vi "Source Current.vi"(7 "Channel Lists":string[](array[string]), 8 "error in (no error)":errorcluster, 10 "current level":dbl format="%_6p", 11 "Instrument Sessions In":refnum<k15>[](array[refnum])) -> (0 "error out":errorcluster, 1 "current measurements":dbl[][](array[numeric]), 2 "voltage measurements":dbl[][](array[numeric]), 3 "Instrument Sessions Out":refnum<k15>[](array[refnum]))   [LabVIEW 2013]
uses:
  <instrlib>/niDCPower/nidcpower.llb/niDCPower Wait For Event - Event.ctl
panel:
  out "Compliance":bool[](array[boolean])
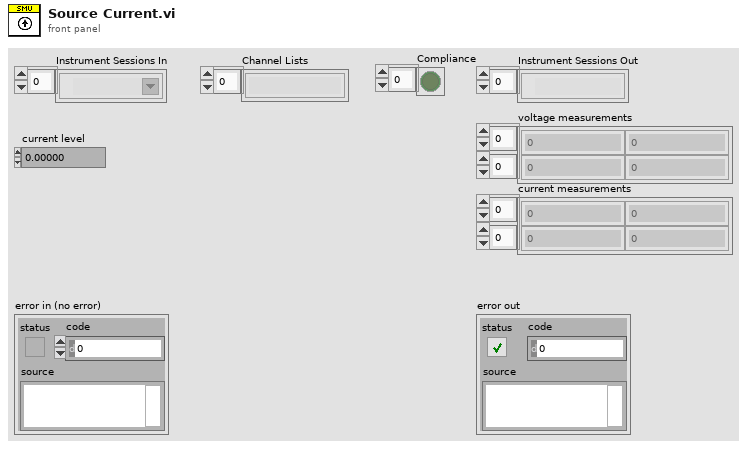
[diagram p1: front panel]
types:
  T1 = typedef "niDCPower Wait For Event - Event.ctl" = i32
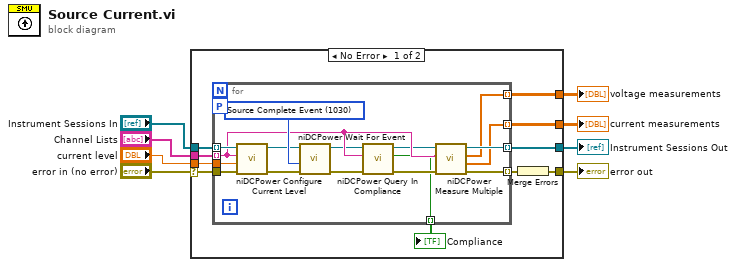
[diagram p0: block diagram]
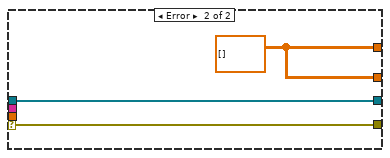
[diagram p2: hidden frame]
diagram:
  n1 = case shown="No Error" "error in (no error)" {
    selector: "error in (no error)" -> [w12 w36]
    tunnel: [w17 w36] -> w8
    tunnel: "Instrument Sessions In" -> [w16 w37]
    tunnel: "Channel Lists" -> [w15 _]
    tunnel: [w14 w37] -> w5
    tunnel: "current level" -> [w13 _]
    tunnel: [w11 w35] -> w2
    tunnel: [w10 w35] -> w1
    frame No Error {
      n2 = for {
        tunnel: w16 -> [w34] mode=indexing
        tunnel: w15 -> [w23] mode=indexing
        tunnel: [w28] -> w14 mode=indexing
        tunnel: [w27] -> w18 mode=indexing
        tunnel: w13 -> [w33]
        tunnel: w12 -> [w32]
        tunnel: [w25] -> w11 mode=indexing
        tunnel: [w26] -> w10 mode=indexing
        tunnel: [w19] -> w9 mode=indexing
        workers-P: _ -> [_]
        w30 = T1 1030 items=["Source Complete Event"=1030, "Measure Complete Event"=1031, "Sequence Iteration Complete Event"=1032, "Sequence Engine Done Event"=1033, "Pulse Complete Event"=1051, "Ready For Pulse Trigger Event"=1052] ("event")
        n3 = call <instrlib>:"niDCPower Configure Current Level.vi"("error in (no error)"=w32, "current level"=w33, "channel name"=w23, "instrument handle"=w34) -> ("error out"=w31:errorcluster, "instrument handle out"=w29:refnum<k15>)  [unwired: 6 in]
        n4 = call <instrlib>:"niDCPower Wait For Event.vi"("error in (no error)"=w31, "event"=w30, "instrument handle"=w29) -> ("error out"=w24:errorcluster, "instrument handle out"=w22:refnum<k15>)  [unwired: 7 in]
        n5 = call <instrlib>:"niDCPower Query In Compliance.vi"("error in (no error)"=w24, "channel name"=w23, "instrument handle"=w22) -> ("error out"=w20:errorcluster, "in compliance?"=w19:bool, "instrument handle out"=w21:refnum<k15>)  [unwired: 6 in]
        n6 = call <instrlib>:"niDCPower Measure Multiple.vi"("error in (no error)"=w20, "channel name"=w23, "instrument handle"=w21) -> ("error out"=w27:errorcluster, "current measurements"=w26:dbl[], "voltage measurements"=w25:dbl[], "instrument handle out"=w28:refnum<k15>)  [unwired: 5 in]
      }
      "Compliance" <- w9
      n7 = Merge Errors(w18) -> (w17:errorcluster)
    }
    frame Error {
      w35 = dbl[][] [] ("voltage measurements")
    }
  }
  "Instrument Sessions Out" <- w5
  "error out" <- w8
  "voltage measurements" <- w2
  "current measurements" <- w1
